vi "Graph - Multi-Y.vi"() -> ()   [LabVIEW 2020, in "Workspace MultiY Graph.lvlib"]
doc: "Sample numeric display item."
uses:
  MultiY Graph LLB.llb/Workspace MultiY Graph.lvlib
  MultiY Graph LLB.llb/cluster_Screen Item Settings.ctl
  MultiY Graph LLB.llb/cluster_Graph Scale Settings.ctl
  MultiY Graph LLB.llb/cluster_Graph Plot Settings.ctl
  NationalInstruments.VeriStand.SystemStorage
  MultiY Graph LLB.llb/XY Top level workspace graph data.ctl
  MultiY Graph LLB.llb/SystemStateRegEventRef.ctl
  MultiY Graph LLB.llb/Target State Info.ctl
  MultiY Graph LLB.llb/Target State.ctl
  MultiY Graph LLB.llb/enum_Display Template Handler Minimal To Widget Msg.ctl
  MultiY Graph LLB.llb/XY Dialog Msg to Control.ctl
  MultiY Graph LLB.llb/XY Dialog Msg Type.ctl
  MultiY Graph LLB.llb/XY Persistent Data.ctl
  MultiY Graph LLB.llb/XY Graph Properties.ctl
  MultiY Graph LLB.llb/XY Plot Properties.ctl
  MultiY Graph LLB.llb/XY Scale Properties.ctl
  MultiY Graph LLB.llb/XY Scale Precision.ctl
  MultiY Graph LLB.llb/XY Scale Format.ctl
  MultiY Graph LLB.llb/UDP Data.ctl
  MultiY Graph LLB.llb/Update Rate.ctl
  MultiY Graph LLB.llb/XY References.ctl
  MultiY Graph LLB.llb/enum_Display Template Handler Minimal To Workspace.ctl
  MultiY Graph LLB.llb/WorkspaceAPI.ctl
  MultiY Graph LLB.llb/SystemStateEventRef.ctl
  MultiY Graph LLB.llb/XY Control Msg to Dialog.ctl
  MultiY Graph LLB.llb/Net Event Data Ref.ctl
  MultiY Graph LLB.llb/Net Event Data.ctl
  MultiY Graph LLB.llb/Net Event.ctl
  MultiY Graph LLB.llb/UDPChannelStreamSession.ctl
  MultiY Graph LLB.llb/UDP Queue Data.ctl
  MultiY Graph LLB.llb/UDP Action State.ctl
  MultiY Graph LLB.llb/Graph Update Queue Data.ctl
  MultiY Graph LLB.llb/Graph Update Action State.ctl
  MultiY Graph LLB.llb/UDP Stream Configuration.ctl
  MultiY Graph LLB.llb/SystemState.ctl
  MultiY Graph LLB.llb/NI_VS Workspace ExecutionAPI.lvlib
  NationalInstruments.VeriStand.ClientAPI
  MultiY Graph LLB.llb/NI_VS UI Tree Alias Browser.lvlib
panel:
  in  "NIVS.Workspace Event":refnum<event-registration>
  in  "NIVS.System Definition Root":refnum<k24>
  in  "NIVS.Gateway IP Address":string
  out "Label":string="Waveform Graph"
  out "Graph":cluster{"X":dbl[], "Y":dbl[]}[](graph)
  in  "Item.Data":T1
  out "Y.Autoscale":bool
  in  "Y.Scale.Once":bool
  in  "Y.Scale.Auto":bool
  out "X.Autoscale":bool
  in  "X.Scale.Once":bool
  in  "X.Scale.Auto":bool
  in  "Legend":bool
  in  "Setup":bool
  in  "Hold":bool
  # "Autoscale X"
  # "Autoscale Y"
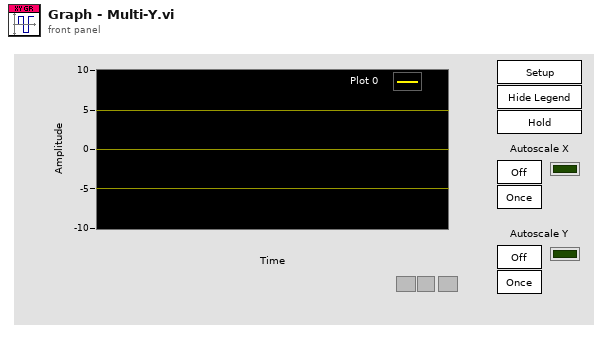
[diagram p1: front panel]
types:
  T1 = typedef "cluster_Screen Item Settings.ctl" = cluster{"Template VI":string, "Position X":i32, "Position Y":i32, "Custom":string, "Show Title Bar":bool, "ID":i32, "Always On Top":bool, "Allow Resize":bool, "Allow Minimize":bool, "Allow Close":bool, "Size to Screen":bool, "Screen.ID":i32, "State":enum16{"Normal", "New"}, "Title":string, "Window Bounds":cluster{"[0]":i16, "[1]":i16, "[2]":i16, "[3]":i16}, "Channel Ref":u64, "Unit":string, "Default Units?":bool, "Flash Limit?":bool, "Color 1":u32, "Color 2":u32, "Color 3":u32, "Color 4":u32, "Bck Color":u32, "Fore Color":u32, "Limit 1":dbl, "Limit 2":dbl, "Limit 3":dbl, "Limit 4":dbl, "Limit Mode 1":i32, "Limit Mode 2":i32, "Limit Mode 3":i32, "Limit Mode 4":i32, "Scale Precision":i32, "Scale Min":dbl, "Scale Max":dbl, "Format":i32, "Precision":i32, "Background Type":i32, "IDs":i32[], "Units":string[], "Labels":string[], "Scale Factor":dbl, "Scale Offset":dbl, "YScale Index":u32[], "XScale":T2, "YScales":T2[], "Plots":T3[], "Update Period":dbl, "History Length":dbl, "My.Ref":refnum<vi>, "Is Control?":bool, "Channel Paths":string[], "Custom Data":variant}
  T2 = typedef "cluster_Graph Scale Settings.ctl" = cluster{"Format":u8, "Precision":u8, "Fit":u8, "Label":string, "Use Default Label":bool, "Label Visible":bool, "Min":dbl, "Max":dbl}
  T3 = typedef "cluster_Graph Plot Settings.ctl" = cluster{"Bar Style":u8, "Fill To":i16, "Fill/PtColor":u32, "Line Style":u8, "Line Width":u8, "Color":u32, "Interp":u8, "Point Style":u8}
  T4 = typedef "Workspace MultiY Graph.lvlib/UDP Action State.ctl" = enum16{"Idle", "Open", "Acquire", "Send", "Close"}
  T5 = typedef "Workspace MultiY Graph.lvlib/UDP Stream Configuration.ctl" = cluster{"net address":u32, "Port":u16, "Channel IDs":i32[], "Packet IDs":i32[], "max packet size":i32, "Graph Buffer Size":i32, "Decimation":i32, "UDP Buffer Size":u32, "ByteOrder":i32}
  T6 = cluster{"connection ID":refnum<k16>, "UDP Stream Configuration":T5, "Graph Buffer":cluster{"X":dbl[], "Y":dbl[]}[], "Dynamic VI Refs":refnum<vi>[]}
  T7 = typedef "Workspace MultiY Graph.lvlib/Graph Update Action State.ctl" = enum16{"Active", "Change Rate", "Inactive"}
  T8 = typedef "Workspace MultiY Graph.lvlib/Graph Update Queue Data.ctl" = cluster{"Graph Update Action State":T7, "Data":variant}
  T9 = typedef "Workspace MultiY Graph.lvlib/UDP Queue Data.ctl" = cluster{"UDP Action State":T4, "Data":variant}
  T10 = typedef "Workspace MultiY Graph.lvlib/XY Top level workspace graph data.ctl" = cluster{"Custom Data":variant, "EventRegs":cluster{"SystemChange":T11, "WorkspaceState":refnum<event-registration>, "Graph":refnum<event-registration>, "Wks&Dialog&Periodic":refnum<event-registration>}, "References":T12, "Persistent Data":T13, "System":cluster{"To Workspace":refnum<user-event>, "From Workspace":refnum<user-event>, "NIVS helper":refnum<vi>, "Gtwy":string, "Root":refnum<k24>, "Workspace":T21, "SystemStateRefs":T22, "Connected?":bool, "FromDialog":refnum<user-event>, "ErrFlag":bool, "New":bool, "ErrState":string, "Save":bool, "Hold":bool, "Periodic":refnum<user-event>, "ToDialog":refnum<user-event>, "DialogEventReg":refnum<event-registration>, "UseSavedWidth":bool, "TreeBrowserEventReg":refnum<event-registration>, "UDPChannelStreamSession":T23, "Valid Channels?":bool, "Update Graph":refnum<user-event>, "UDP Queue":refnum<queue>, "Graph Update Queue":refnum<queue>}, "GraphData":cluster{"X":dbl[], "Y":dbl[]}[], "UDP Stream Active?":bool}
  T11 = typedef "NI_VS Workspace ExecutionAPI.lvlib/SystemStateRegEventRef.ctl" = refnum<event-registration>
  T12 = typedef "Workspace MultiY Graph.lvlib/XY References.ctl" = cluster{"X.Scale.Auto":refnum<vi>, "Y.Scale.Auto":refnum<vi>, "X.Scale.Once":refnum<vi>, "Y.Scale.Once":refnum<vi>, "LegendVis":refnum<vi>, "Graph":refnum<vi>}
  T13 = typedef "Workspace MultiY Graph.lvlib/XY Persistent Data.ctl" = cluster{"Label":string, "Graph Props":T14, "UDP Data":T19}
  T14 = typedef "Workspace MultiY Graph.lvlib/XY Graph Properties.ctl" = cluster{"Plots":T15[], "Legend:Number of Rows":u32, "Scale Properties":T16, "Legend:Visible":bool, "BgColor":u32, "Last Plot Width":u32, "Resize":bool}
  T15 = typedef "Workspace MultiY Graph.lvlib/XY Plot Properties.ctl" = cluster{"Bar Plot Style":u8, "Digital Line Style":u8, "Digital Transition Location":u8, "Digital Transition Type":u8, "Fill To":i16, "Fill/Point Color":u32, "Label Format":u8, "Line Style":u8, "Line Width":u8, "Plot Color":u32, "Plot Interpolation":u8, "Point Style":u8, "Visible":bool, "X Scale Index":u32, "Y Scale Index":u32}
  T16 = typedef "Workspace MultiY Graph.lvlib/XY Scale Properties.ctl" = cluster{"X.Auto":bool, "X.Min":dbl, "X.Max":dbl, "X.IgnoreTS":bool, "X.Precision":T17, "X.Label:":string, "X.LabelVis":bool, "X.DefLabel":bool, "Y.Auto":bool, "Y.Min":dbl, "Y.Max":dbl, "Y.Format":T18, "Y.Precision:":T17, "Y.Label:":string, "Y.LabelVis":bool, "Y.DefLabel":bool, "X.Format":T18}
  T17 = typedef "Workspace MultiY Graph.lvlib/XY Scale Precision.ctl" = u8
  T18 = typedef "Workspace MultiY Graph.lvlib/XY Scale Format.ctl" = u8
  T19 = typedef "Workspace MultiY Graph.lvlib/UDP Data.ctl" = cluster{"Decimation":i32, "UDP Buffer Size":u32, "History Length":dbl, "Update Rate":T20, "Channel Paths":string[], "Channel Names":string[]}
  T20 = typedef "Workspace MultiY Graph.lvlib/Update Rate.ctl" = enum8{"15 Hz", "10 Hz", "5 Hz", "4 Hz", "3 Hz", "2 Hz", "1 Hz", "0.5 Hz"}
  T21 = typedef "NI_VS Workspace ExecutionAPI.lvlib/WorkspaceAPI.ctl" = refnum<k24>
  T22 = typedef "NI_VS Workspace ExecutionAPI.lvlib/SystemStateEventRef.ctl" = cluster{"CustDatRef":refnum<user-event>, "EvtRef":refnum<k27>, "Target State User Event":refnum<user-event>}
  T23 = typedef "NI_VS Workspace ExecutionAPI.lvlib/UDPChannelStreamSession.ctl" = refnum<k24>
  T24 = cluster{"connection ID":refnum<k16>, "UDP Stream Configuration out":T5, "Array Out":cluster{"X":dbl[], "Y":dbl[]}[], "Dynamic VI Refs":refnum<vi>[]}
  T25 = typedef "Workspace MultiY Graph.lvlib/XY Control Msg to Dialog.ctl" = enum16{"Stop", "Connecting", "Disconnecting"}
  T26 = typedef "enum_Display Template Handler Minimal To Workspace.ctl" = cluster{"Operation":enum16{"SetCustomData", "DeleteItem"}, "Data":variant}
  T27 = cluster{"SystemChange":T11, "WorkspaceState":refnum<event-registration>, "Graph":refnum<event-registration>, "Wks&Dialog&Periodic":refnum<event-registration>}
  T28 = typedef "enum_Display Template Handler Minimal To Widget Msg.ctl" = enum16{"Stop", "LaunchConfigDialog"}
  T29 = typedef "Workspace MultiY Graph.lvlib/XY Dialog Msg Type.ctl" = enum16{"Update", "Delete"}
  T30 = typedef "NI_VS Workspace ExecutionAPI.lvlib/SystemState.ctl" = u8
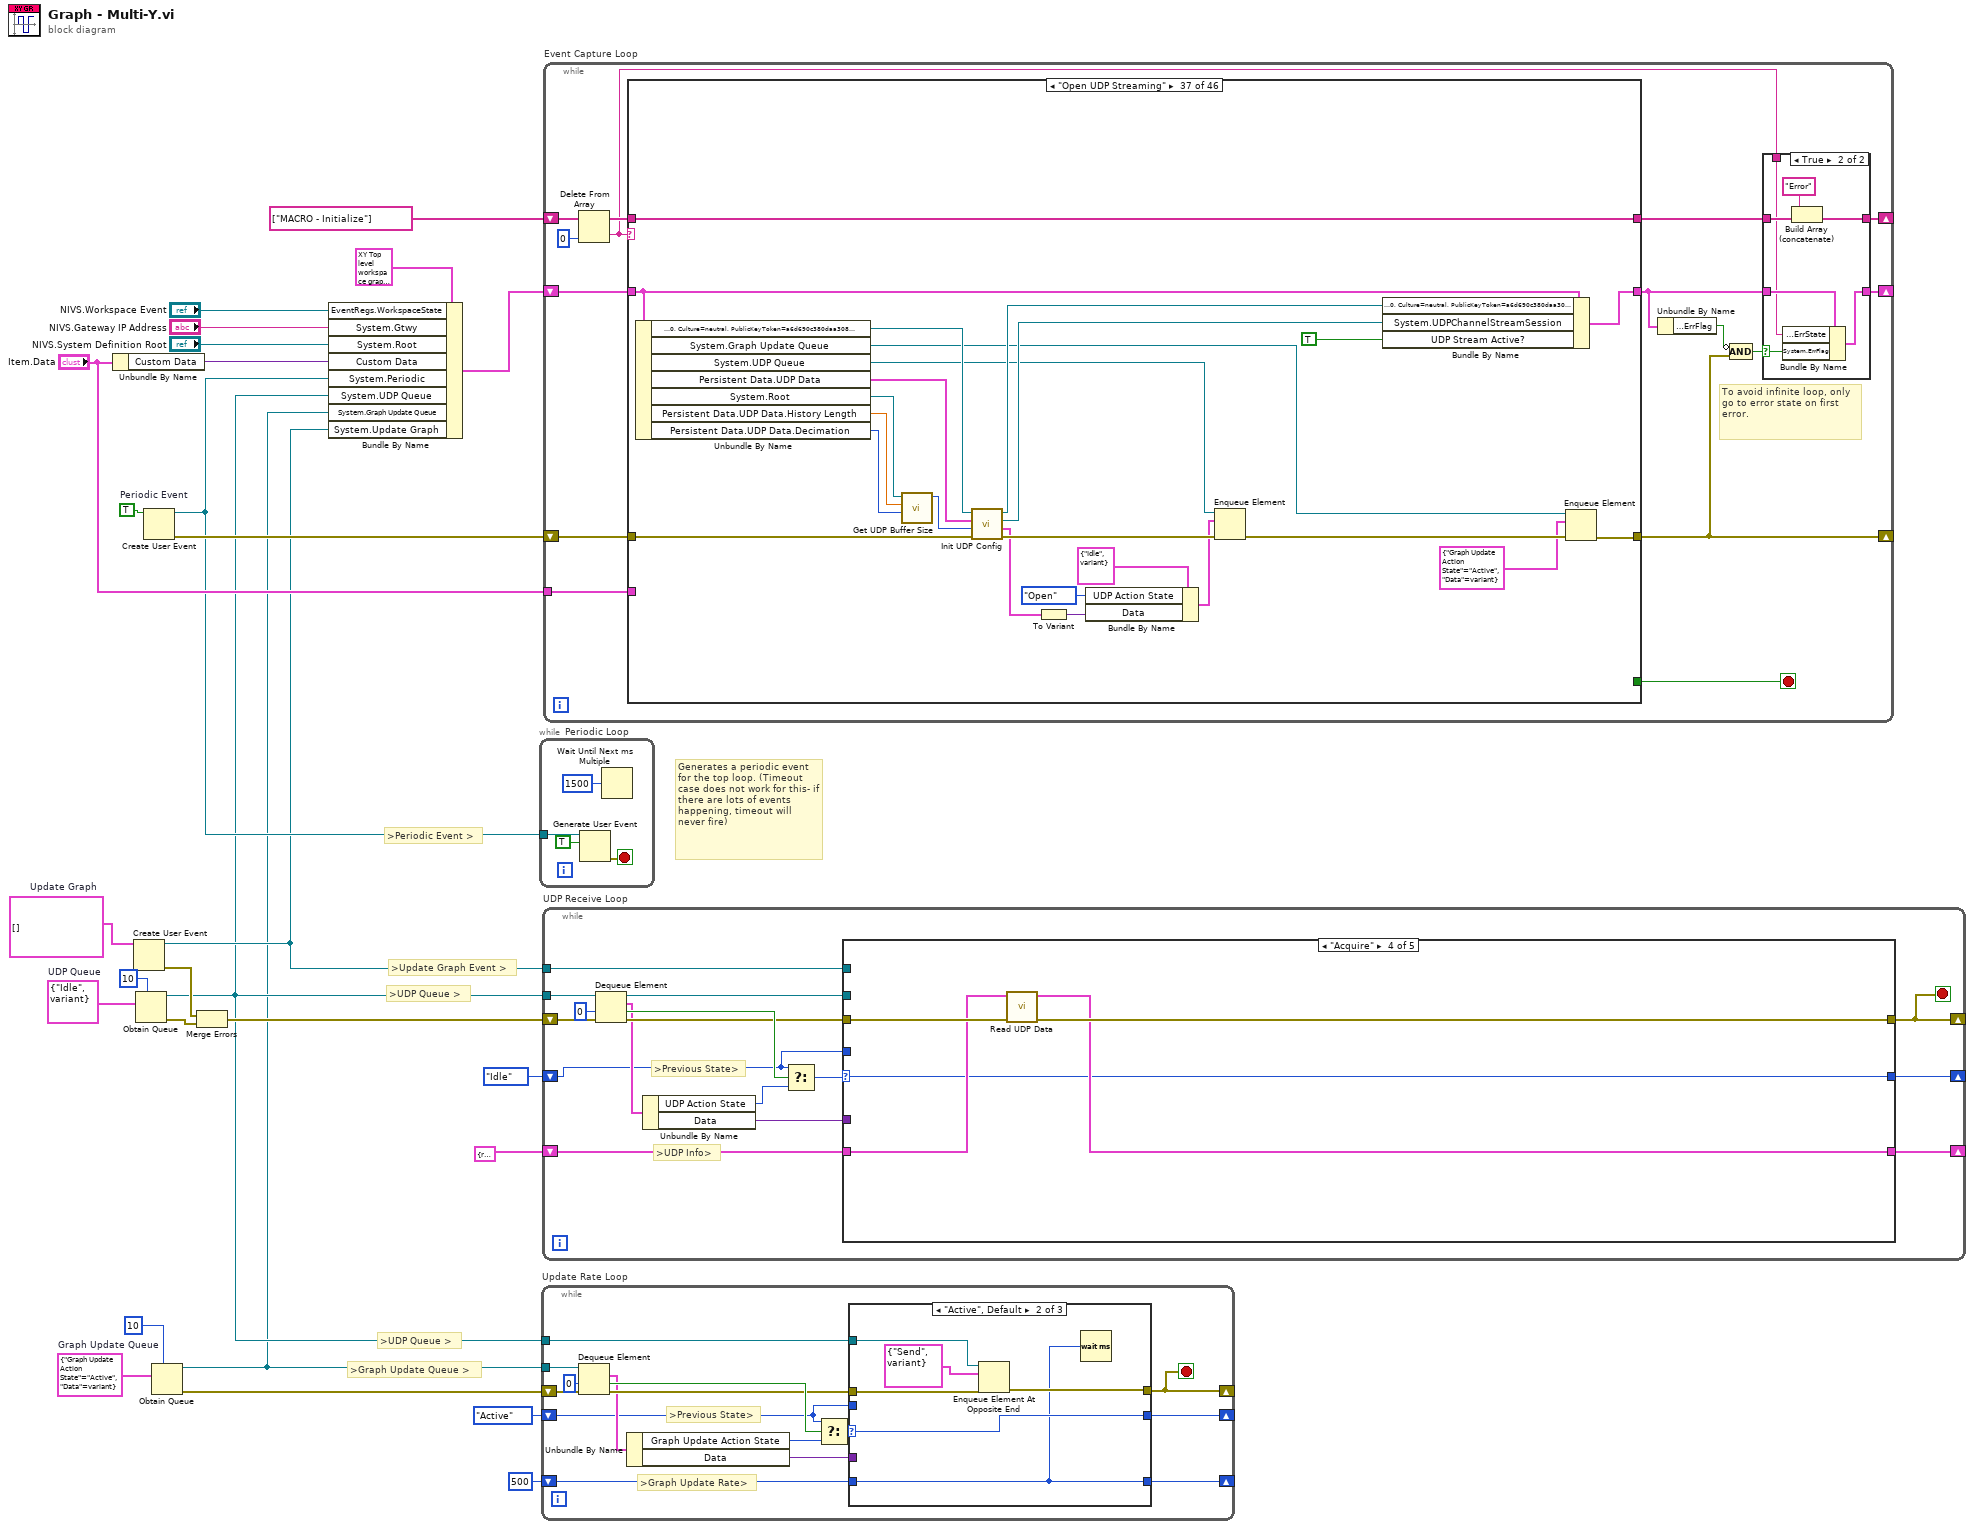
[diagram p0: block diagram]
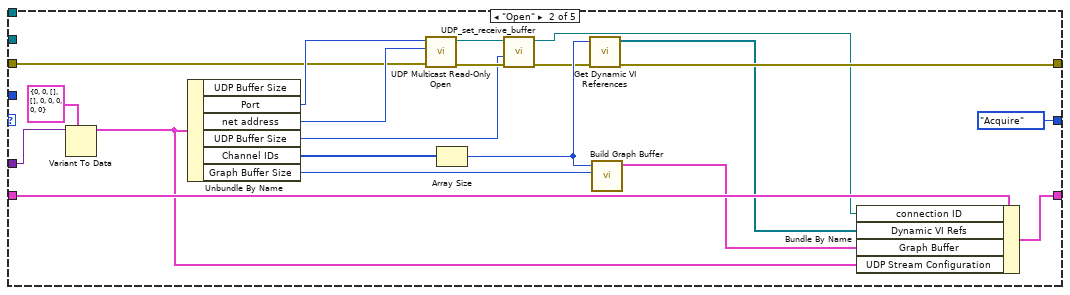
[diagram p3: hidden frame]
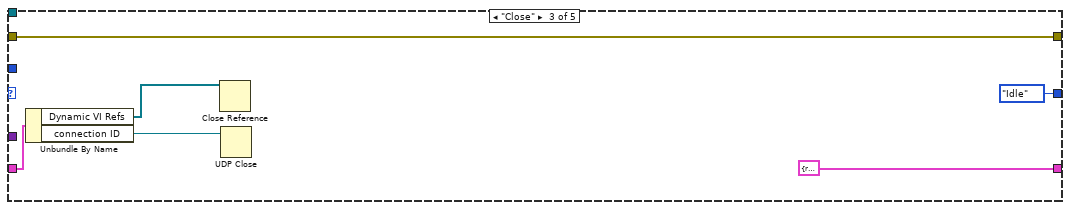
[diagram p4: hidden frame]
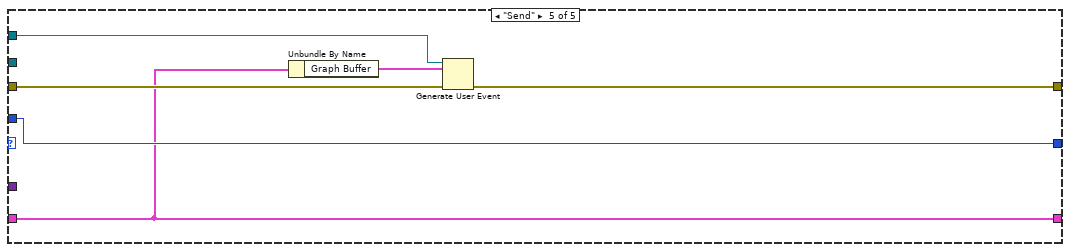
[diagram p5: hidden frame]
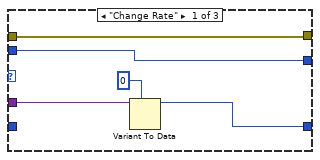
[diagram p6: hidden frame]
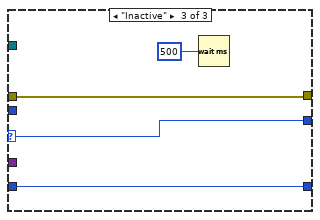
[diagram p7: hidden frame]
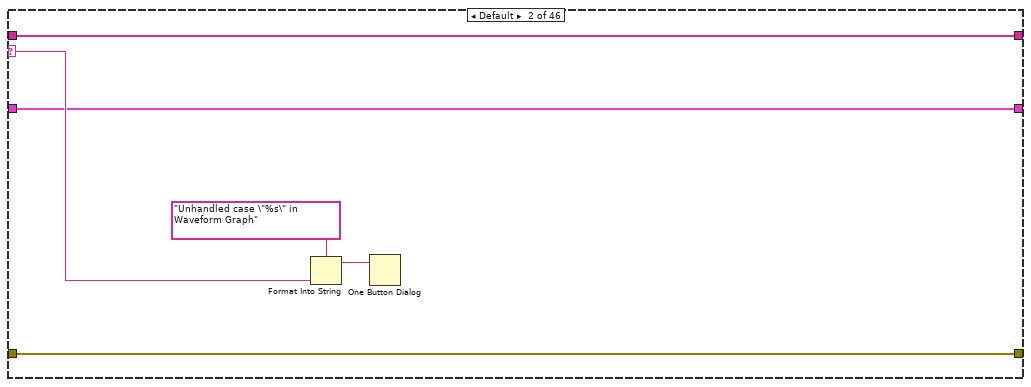
[diagram p10: hidden frame]
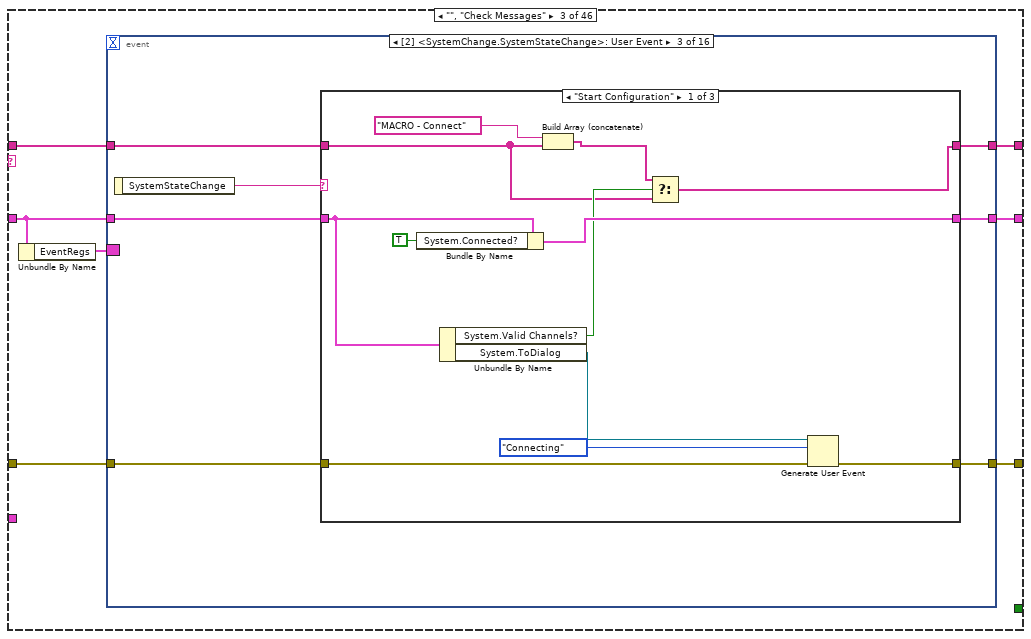
[diagram p11: hidden frame]
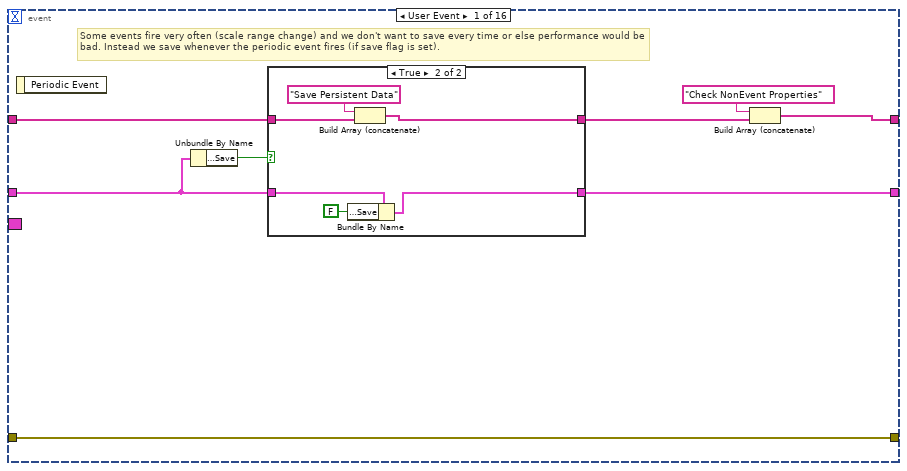
[diagram p12: hidden frame]
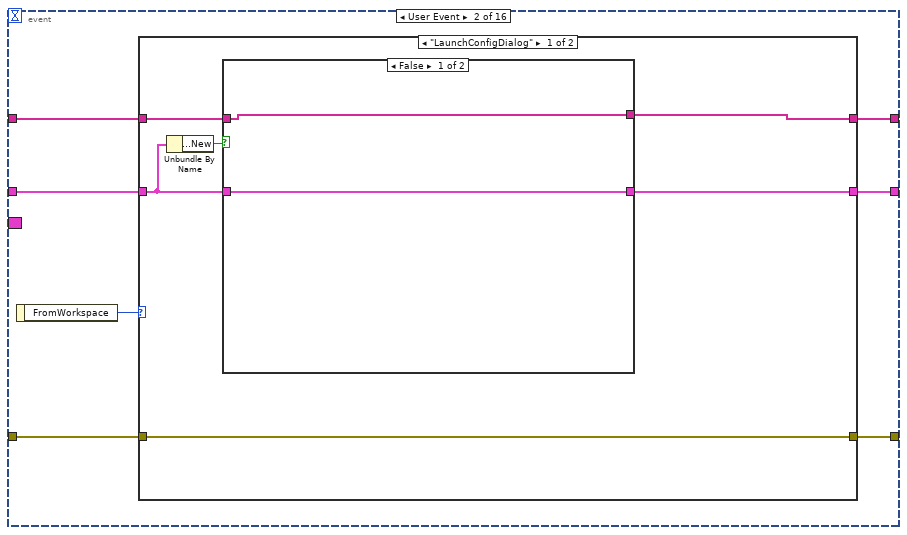
[diagram p14: hidden frame]
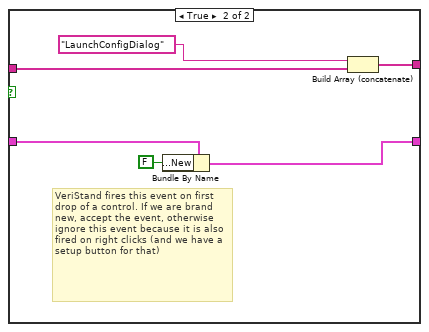
[diagram p15: hidden frame]
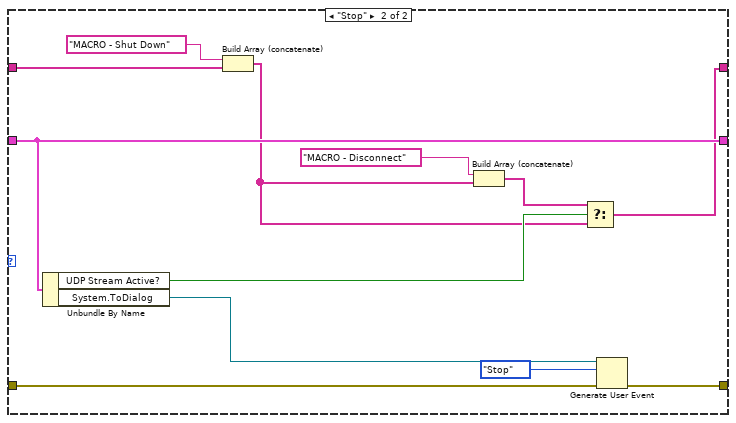
[diagram p16: hidden frame]
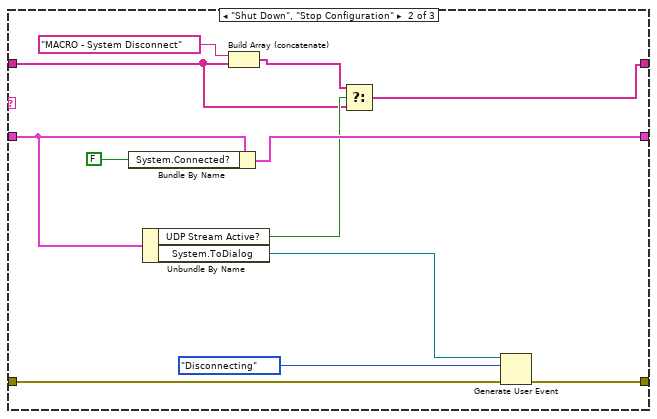
[diagram p17: hidden frame]
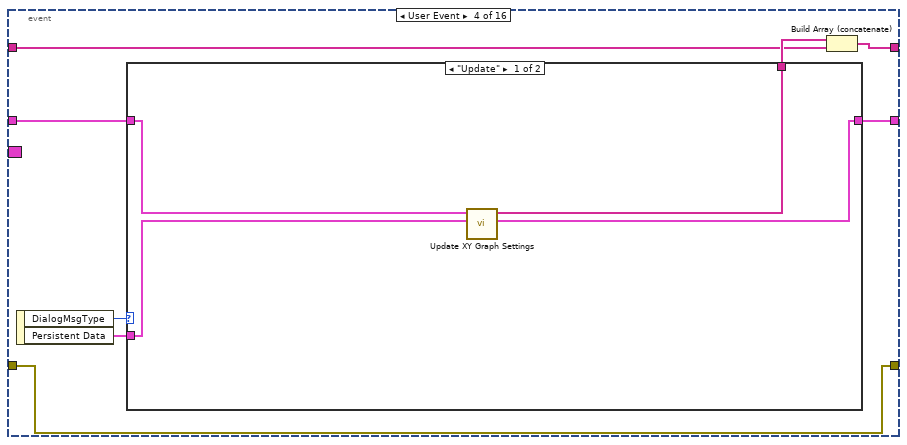
[diagram p19: hidden frame]
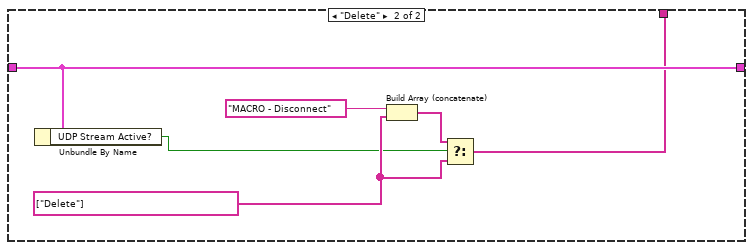
[diagram p20: hidden frame]
diagram:
  w13 = T8 {"Graph Update Action State"=enum."Active", "Data"=variant}  # Graph Update Queue
  w15 = T9 {"UDP Action State"=enum."Idle", "Data"=variant}  # UDP Queue
  w16 = cluster{"X":dbl[], "Y":dbl[]}[] []  # Update Graph
  w18 = TRUE  # Periodic Event
  # ">UDP Queue >"
  # ">Update Graph Event >"
  # ">Periodic Event >"
  # ">Graph Update Queue >"
  # ">UDP Queue >"
  # "Generates a periodic event for the top loop. (Timeout case does not work for this- if there are lots of events happening, timeout will never fire)"
  n1 = Unbundle By Name("Item.Data") -> ("Custom Data"=w26:variant)
  n2 = Create User Event(user event datatype=w16) -> (user event=w14:refnum<user-event>, error out=w9:errorcluster)  [unwired: 1 in]
  n3 = Obtain Queue(max queue size (-1, unlimited)=10, element data type=w15) -> (queue out=w6:refnum<queue>, error out=w10:errorcluster)  [unwired: 3 in, 1 out]
  n4 = Create User Event(user event datatype=w18) -> (user event=w17:refnum<user-event>, error out=w19:errorcluster)  [unwired: 1 in]
  n5 = Obtain Queue(max queue size (-1, unlimited)=10, element data type=w13) -> (queue out=w3:refnum<queue>, error out=w11:errorcluster)  [unwired: 3 in, 1 out]
  n6 = Merge Errors(w9, w10) -> (w8:errorcluster)
  n7 = Bundle By Name(cluster=T10 {"Custom Data"=variant, "EventRegs"={"SystemChange"=refnum, "WorkspaceState"=refnum, "Graph"=refnum, "Wks&Dialog&Periodic"=refnum}, "References"={"X.Scale.Auto"=refnum, "Y.Scale.Auto"=refnum, "X.Scale.Once"=refnum, "Y.Scale.Once"=refnum, "LegendVis"=refnum, "Graph"=refnum}, "Persistent Data"={"Label"="", "Graph Props"={"Plots"=[], "Legend:Number of Rows"=0, "Scale Properties"={"X.Auto"=FALSE, "X.Min"=0.0, "X.Max"=0.0, "X.IgnoreTS"=FALSE, "X.Precision"=0, "X.Label:"="", "X.LabelVis"=FALSE, "X.DefLabel"=FALSE, "Y.Auto"=FALSE, "Y.Min"=0.0, "Y.Max"=0.0, "Y.Format"=0, "Y.Precision:"=0, "Y.Label:"="", "Y.LabelVis"=FALSE, "Y.DefLabel"=FALSE, "X.Format"=0}, "Legend:Visible"=FALSE, "BgColor"=0, "Last Plot Width"=0, "Resize"=FALSE}, "UDP Data"={"Decimation"=0, "UDP Buffer Size"=0, "History Length"=0.0, "Update Rate"=enum."15 Hz", "Channel Paths"=[], "Channel Names"=[]}}, "System"={"To Workspace"=refnum, "From Workspace"=refnum, "NIVS helper"=refnum, "Gtwy"="", "Root"=refnum, "Workspace"=refnum, "SystemStateRefs"={"CustDatRef"=refnum, "EvtRef"=refnum, "Target State User Event"=refnum}, "Connected?"=FALSE, "FromDialog"=refnum, "ErrFlag"=FALSE, "New"=FALSE, "ErrState"="", "Save"=FALSE, "Hold"=FALSE, "Periodic"=refnum, "ToDialog"=refnum, "DialogEventReg"=refnum, "UseSavedWidth"=FALSE, "TreeBrowserEventReg"=refnum, "UDPChannelStreamSession"=refnum, "Valid Channels?"=FALSE, "Update Graph"=refnum, "UDP Queue"=refnum, "Graph Update Queue"=refnum}, "GraphData"=[], "UDP Stream Active?"=FALSE} ("Waveform Graph Data"), "EventRegs.WorkspaceState"="NIVS.Workspace Event", "System.Gtwy"="NIVS.Gateway IP Address", "System.Root"="NIVS.System Definition Root", "Custom Data"=w26, "System.Periodic"=w17, "System.UDP Queue"=w6, "System.Graph Update Queue"=w3, "System.Update Graph"=w14) -> (w21:T10)
  n8 = while "Periodic Loop" {
    tunnel: w17 -> [w30]
    stop <- w29 stop-if-true
    n9 = Generate User Event(user event=w30, event data cluster=TRUE ("event data")) -> (error out=w29:errorcluster)  [unwired: 2 in, 1 out]
    n10 = Wait Until Next ms Multiple(millisecond multiple=u32 1500) -> ()  [unwired: 1 out]
  }
  n11 = while "Update Rate Loop" {
    tunnel: w3 -> [w45]
    shift-right: [w39] -> _
    shift-left: w11 -> [w46]
    shift-right: [w41] -> _
    shift-left: Graph_Update_Action_State."Active" ("Graph Update Action State") -> [w33]
    tunnel: w6 -> [w38]
    shift-right: [w34] -> _
    shift-left: u32 500 ("element") -> [w32]
    stop <- w39 stop-if-true
    # ">Previous State>"
    # ">Graph Update Rate>"
    n12 = Dequeue Element(queue=w45, timeout in ms (-1)=0, error in (no error)=w46) -> (element=w37:T8, timed out?=w43:bool, error out=w40:errorcluster)  [unwired: 1 out]
    n13 = Unbundle By Name(w37) -> ("Graph Update Action State"=w36:T7, "Data"=w35:variant)
    n14 = Select(t=w33, s=w43, f=w36) -> (s? t:f=w42:T7)
    n15 = case shown="\"Active\", Default" w42 {
      selector: w42 -> [_ w57 w61]
      tunnel: [w47 w57 w61] -> w41
      tunnel: w40 -> [w51 w56 w60]
      tunnel: [w51 w53 w60] -> w39
      tunnel: w38 -> [_ w55 _]
      tunnel: w35 -> [w50 _ _]
      tunnel: [w48 w52 w58] -> w34
      tunnel: w33 -> [w47 _ _]
      tunnel: w32 -> [_ w52 w58]
      frame "Change Rate" {
        n16 = Variant To Data(type=u32 0 ("element"), Variant=w50) -> (data=w48:u32)  [unwired: 1 in, 1 out]
      }
      frame "Active", Default {
        n17 = Enqueue Element At Opposite End(queue=w55, element=T9 {"UDP Action State"=enum."Send", "Data"=variant} ("notification"), error in (no error)=w56) -> (error out=w53:errorcluster)  [unwired: 1 in, 2 out]
        n18 = Wait (ms)(milliseconds to wait=w52) -> ()  [unwired: 1 out]
      }
      frame "Inactive" {
        n19 = Wait (ms)(milliseconds to wait=u32 500) -> ()  [unwired: 1 out]
      }
    }
  }
  n20 = while "UDP Receive Loop" {
    tunnel: w6 -> [w76]
    shift-right: [w70] -> _
    shift-left: w8 -> [w77]
    shift-right: [w72] -> _
    shift-left: UDP_Action_State."Idle" ("UDP Action State") -> [w63]
    shift-right: [w68] -> _
    shift-left: T6 {"connection ID"=refnum, "UDP Stream Configuration"={"net address"=0, "Port"=0, "Channel IDs"=[], "Packet IDs"=[], "max packet size"=0, "Graph Buffer Size"=0, "Decimation"=0, "UDP Buffer Size"=0, "ByteOrder"=0}, "Graph Buffer"=[], "Dynamic VI Refs"=[]} -> [w69]
    tunnel: w14 -> [w62]
    stop <- w70 stop-if-true
    # ">UDP Info>"
    # ">Previous State>"
    n21 = Dequeue Element(queue=w76, timeout in ms (-1)=0, error in (no error)=w77) -> (queue out=w75:refnum<queue>, element=w65:T9, timed out?=w73:bool, error out=w71:errorcluster)
    n22 = Unbundle By Name(w65) -> ("UDP Action State"=w66:T4, "Data"=w64:variant)
    n23 = Select(t=w63, s=w73, f=w66) -> (s? t:f=w67:T4)
    n24 = case shown="\"Acquire\"" w67 {
      selector: w67 -> [w80 _ _ w107 _]
      tunnel: w71 -> [w79 w88 w102 w111 w114]
      tunnel: [w79 w93 w102 w110 w113] -> w70
      tunnel: w75 -> [_ _ _ _ _]
      tunnel: [w80 UDP_Action_State."Acquire" ("UDP Action State") UDP_Action_State."Idle" ("UDP Action State") w107 w117] -> w72
      tunnel: w69 -> [w78 w97 w105 w109 w112]
      tunnel: [w78 w96 T24 {"connection ID"=refnum, "UDP Stream Configuration out"={"net address"=0, "Port"=0, "Channel IDs"=[], "Packet IDs"=[], "max packet size"=0, "Graph Buffer Size"=0, "Decimation"=0, "UDP Buffer Size"=0, "ByteOrder"=0}, "Array Out"=[], "Dynamic VI Refs"=[]} w108 w112] -> w68
      tunnel: w64 -> [_ w91 _ _ _]
      tunnel: w63 -> [_ _ _ _ w117]
      tunnel: w62 -> [_ _ _ _ w115]
      frame "Idle", Default {
      }
      frame "Open" {
        n25 = Variant To Data(type=T5 {"net address"=0, "Port"=0, "Channel IDs"=[], "Packet IDs"=[], "max packet size"=0, "Graph Buffer Size"=0, "Decimation"=0, "UDP Buffer Size"=0, "ByteOrder"=0} ("UDP Stream Configuration out"), Variant=w91) -> (data=w89:T5)  [unwired: 1 in, 1 out]
        n26 = Unbundle By Name(w89) -> ("Port"=w100:u16, "net address"=w99:u32, "UDP Buffer Size"=w81:u32, "Channel IDs"=w95:i32[], "Graph Buffer Size"=w98:i32)  [unwired: 1 out]
        n27 = call "UDP Multicast Read-Only Open.vi"("error in (no error)"=w88, "multicast addr"=w99, "port"=w100) -> ("error out"=w85:errorcluster, "connection ID"=w84:refnum<k16>)  [unwired: 6 in, 1 out]
        n28 = Array Size(array=w95) -> (size(s)=w94:i32)
        n29 = call "UDP_set_receive_buffer.vi"("error in (no error)"=w85, "Receive Buffer Size"=w81, "connection ID"=w84) -> ("error out"=w82:errorcluster, "connection ID out"=w83:refnum<k16>)  [unwired: 6 in]
        n30 = call "Get Dynamic VI References.vi"("error in (no error)"=w82, "Channel Count"=w94) -> ("error out"=w93:errorcluster, "Dynamic VI References"=w92:refnum<vi>[])  [unwired: 8 in]
        n31 = call "Build Graph Buffer.vi"("Graph Buffer Size"=w98, "Channel Count"=w94) -> ("Graph Buffer out"=w86:cluster{dbl[], dbl[]}[])  [unwired: 9 in]
        n32 = Bundle By Name(cluster=w97, "connection ID"=w83, "Dynamic VI Refs"=w92, "Graph Buffer"=w86, "UDP Stream Configuration"=w89) -> (w96:T6)
      }
      frame "Close" {
        n33 = Unbundle By Name(w105) -> ("Dynamic VI Refs"=w104:refnum<vi>[], "connection ID"=w103:refnum<k16>)
        n34 = Close Reference(reference=w104) -> ()  [unwired: 1 in, 1 out]
        n35 = UDP Close(connection ID=w103) -> ()  [unwired: 1 in, 2 out]
      }
      frame "Acquire" {
        n36 = call "Read UDP Data.vi"("error in (no error)"=w111, "UDP Cluster in"=w109) -> ("error out"=w110:errorcluster, "UDP Cluster out"=w108:T6)  [unwired: 8 in]
      }
      frame "Send" {
        n37 = Unbundle By Name(w112) -> ("Graph Buffer"=w116:cluster{"X":dbl[], "Y":dbl[]}[])
        n38 = Generate User Event(user event=w115, event data cluster=w116, error in=w114) -> (error out=w113:errorcluster)  [unwired: 1 in, 1 out]
      }
    }
  }
  n39 = while "Event Capture Loop" {
    shift-right: [w126] -> _
    shift-left: string[] ["MACRO - Initialize"] -> [w132]
    shift-right: [w119] -> _
    shift-left: w19 -> [w125]
    shift-right: [w123] -> _
    shift-left: w21 -> [w128]
    tunnel: "Item.Data" -> [w127]
    stop <- w130 stop-if-true
    # "To avoid infinite loop, only go to error state on first error."
    n40 = Delete From Array(array=w132, index=0) -> (deleted portion=w118:string, array with subset deleted=w131:string[])  [unwired: 1 in]
    n41 = case shown="\"Open UDP Streaming\"" w118 {
      selector: w118 -> [_ w149 _ _ _ _ _ _ _ _ _ _ _ _ _ _ _ _ _ _ _ _ _ _ _ _ _ _ _ _ _ _ _ _ _ _ _ _ _ _ _ _ _ _ _ _]
      tunnel: [w142 w145 w157 string[] ["MACRO - Disconnect"] w440 w448 w450 w459 w460 w470 w482 w485 w489 w507 w530 w541 w552 w585 w619 w635 w656 w681 w689 w699 w700 w704 w707 w714 w718 w723 w728 w733 w739 w755 w769 w772 w796 w797 w806 w809 w818 w823 w838 w847 w871 w889] -> w129
      tunnel: w131 -> [w142 w145 w156 _ w440 w448 w450 w459 w460 w470 w482 w485 w489 w507 w530 w541 w552 w585 w619 w635 w656 w681 w689 w699 w700 w704 w708 w715 w721 w724 w729 w736 w739 w755 w769 w772 w796 w797 w806 w809 w818 w827 w838 w846 w871 w889]
      tunnel: [_ _ _ _ _ _ _ _ _ _ _ _ _ _ _ _ _ _ _ _ _ _ _ _ TRUE _ _ _ _ _ _ _ _ _ _ _ _ _ _ _ _ _ _ _ _ _] -> w130
      tunnel: w125 -> [w144 w147 w154 w424 w436 w447 w452 w453 w466 w469 w473 w484 w488 w506 w529 w540 w547 w584 w618 w632 w658 w667 w688 w692 w702 w706 w711 w716 w720 w726 w731 w735 w738 w752 w766 w771 w794 w799 w805 w808 w821 w832 w837 w852 w869 w885]
      tunnel: [w144 w147 w153 errorcluster {"status"=FALSE, "code"=0, "source"=""} ("error constant") w439 w444 w451 w453 w464 w469 w472 w484 w488 w495 w517 w537 w548 w576 w615 w633 w658 w674 w685 w691 w702 w706 w711 w716 w720 w726 w731 w735 w738 w741 w758 w771 w787 w799 w800 w810 w821 w831 w837 w851 w865 w886] -> w119
      tunnel: w128 -> [w143 w146 w152 w426 w433 w446 w449 w458 w467 w468 w481 w483 w487 w499 w522 w539 w551 w583 w617 w634 w657 w684 w687 w698 w701 w705 w710 w713 w719 w725 w730 w734 w737 w751 w765 w770 w791 w798 w802 w807 w820 w829 w836 w842 w870 w879]
      tunnel: [w143 w146 w155 w426 w432 w445 w449 w457 w467 w468 w481 w483 w487 w498 w521 w539 w551 w583 w617 w634 w657 w684 w687 w698 w701 w705 w710 w713 w719 w725 w730 w734 w737 w750 w764 w770 w790 w798 w804 w811 w819 w828 w835 w844 w870 w873] -> w122
      tunnel: w127 -> [_ _ _ _ _ _ _ _ _ _ _ _ _ _ _ _ _ _ _ _ _ _ _ _ _ _ _ _ _ _ _ _ _ _ _ _ _ _ _ _ _ _ _ _ _ w875]
      frame "<------------------ System ------------------>" {
      }
      frame Default {
        n42 = Format Into String(format string="Unhandled case \"%s\" in Waveform Graph", w149) -> (resulting string=w150:string)  [unwired: 2 in, 1 out]
        n43 = One Button Dialog(message=w150) -> ()  [unwired: 1 in, 1 out]
      }
      frame "", "Check Messages" {
        n44 = Unbundle By Name(w152) -> ("EventRegs"=w151:T27)
        n45 = event shown="[2] <SystemChange.SystemStateChange>: User Event" {
          selector: w151 -> [_ _ _ _ _ _ _ _ _ _ _ _ _ _ _ _]
          dyn-events: _ -> [_ _ _ _ _ _ _ _ _ _ _ _ _ _ _ _]
          timeout: _ -> [_ _ _ _ _ _ _ _ _ _ _ _ _ _ _ _]
          tunnel: [w158 w174 w213 w246 w265 w286 w293 w300 w306 w316 w323 w335 w343 w354 w367 w380] -> w157
          tunnel: w156 -> [w165 w178 w212 w247 w264 w286 w293 w302 w314 w321 w328 w338 w349 w360 w367 w379]
          tunnel: [w164 w175 w211 w245 w263 w284 w289 w304 w308 w318 w325 w337 w341 w352 w362 w381] -> w155
          tunnel: w152 -> [w162 w176 w210 w244 w262 w281 w292 w304 w310 w319 w326 w331 w346 w357 w365 w382]
          tunnel: w154 -> [w161 w180 w208 w241 w260 w282 w291 w303 w313 w320 w327 w333 w348 w359 w366 w383]
          tunnel: [w161 w177 w209 w241 w261 w282 w290 w303 w312 w320 w327 w332 w347 w358 w366 w384] -> w153
          event User Event {
            # "Some events fire very often (scale range change) and we don't want to save every time or else performance would be bad. Instead we save whenever the periodic event fires (if save flag is set)."
            n46 = event-data() -> ()  [unwired: 1 in, 1 out]
            n47 = Unbundle By Name(w162) -> ("System.Save"=w163:bool)
            n48 = case shown="True" w163 {
              tunnel: w165 -> [w167 w170]
              tunnel: [w167 w168] -> w160
              tunnel: [w166 w171] -> w164
              tunnel: w162 -> [w166 w173]
              frame False {
              }
              frame True {
                n49 = Bundle By Name(cluster=w173, "System.Save"=FALSE) -> (w171:T10)
                n50 = Build Array (concatenate)("Save Persistent Data", w170) -> (w168:string[])
              }
            }
            n51 = Build Array (concatenate)("Check NonEvent Properties", w160) -> (w158:string[])
          }
          event User Event {
            n52 = event-data() -> ("FromWorkspace"=w179:T28)  [unwired: 1 in]
            n53 = case shown="\"LaunchConfigDialog\"" w179 {
              tunnel: w180 -> [w186 w203]
              tunnel: w178 -> [w185 w206]
              tunnel: [w186 w202] -> w177
              tunnel: w176 -> [w182 w204]
              tunnel: [w181 w204] -> w175
              tunnel: [w184 w195] -> w174
              frame "LaunchConfigDialog" {
                n54 = Unbundle By Name(w182) -> ("System.New"=w183:bool)
                n55 = case shown="False" w183 {
                  tunnel: w185 -> [w187 w194]
                  tunnel: [w187 w192] -> w184
                  tunnel: w182 -> [w188 w191]
                  tunnel: [w188 w190] -> w181
                  frame False {
                  }
                  frame True {
                    # "VeriStand fires this event on first drop of a control. If we are brand new, accept the event, otherwise ignore this event because it is also fired on right clicks (and we have a setup button for that)"
                    n56 = Bundle By Name(cluster=w191, "System.New"=FALSE) -> (w190:T10)
                    n57 = Build Array (concatenate)("LaunchConfigDialog", w194) -> (w192:string[])
                  }
                }
              }
              frame "Stop" {
                n58 = Unbundle By Name(w204) -> ("UDP Stream Active?"=w197:bool, "System.ToDialog"=w201:refnum<user-event>)
                n59 = Build Array (concatenate)("MACRO - Shut Down", w206) -> (w196:string[])
                n60 = Build Array (concatenate)("MACRO - Disconnect", w196) -> (w198:string[])
                n61 = Select(t=w198, s=w197, f=w196) -> (s? t:f=w195:string[])
                n62 = Generate User Event(user event=w201, event data cluster=XY_Control_Msg_to_Dialog."Stop" ("event data"), error in=w203) -> (error out=w202:errorcluster)  [unwired: 1 in, 1 out]
              }
            }
          }
          event User Event {
            n63 = event-data() -> ("SystemStateChange"=w207:string)  [unwired: 1 in]
            n64 = case shown="\"Start Configuration\"" w207 {
              tunnel: [w214 w226 w240] -> w213
              tunnel: w212 -> [w216 w227 w240]
              tunnel: [w224 w236 w239] -> w211
              tunnel: w210 -> [w219 w230 w239]
              tunnel: [w220 w231 w238] -> w209
              tunnel: w208 -> [w221 w232 w238]
              frame "Start Configuration" {
                n65 = Bundle By Name(cluster=w219, "System.Connected?"=TRUE) -> (w224:T10)
                n66 = Unbundle By Name(w219) -> ("System.Valid Channels?"=w217:bool, "System.ToDialog"=w223:refnum<user-event>)
                n67 = Build Array (concatenate)("MACRO - Connect", w216) -> (w215:string[])
                n68 = Select(t=w215, s=w217, f=w216) -> (s? t:f=w214:string[])
                n69 = Generate User Event(user event=w223, event data cluster=XY_Control_Msg_to_Dialog."Connecting" ("event data"), error in=w221) -> (error out=w220:errorcluster)  [unwired: 1 in, 1 out]
              }
              frame "Shut Down", "Stop Configuration" {
                n70 = Bundle By Name(cluster=w230, "System.Connected?"=FALSE) -> (w236:T10)
                n71 = Unbundle By Name(w230) -> ("UDP Stream Active?"=w229:bool, "System.ToDialog"=w234:refnum<user-event>)
                n72 = Build Array (concatenate)("MACRO - System Disconnect", w227) -> (w228:string[])
                n73 = Select(t=w228, s=w229, f=w227) -> (s? t:f=w226:string[])
                n74 = Generate User Event(user event=w234, event data cluster=XY_Control_Msg_to_Dialog."Disconnecting" ("event data"), error in=w232) -> (error out=w231:errorcluster)  [unwired: 1 in, 1 out]
              }
              frame Default {
              }
            }
          }
          event User Event {
            n75 = event-data() -> ("DialogMsgType"=w242:T29, "Persistent Data"=w243:T13)  [unwired: 1 in]
            n76 = case shown="\"Update\"" w242 {
              tunnel: w244 -> [w251 w258]
              tunnel: [w252 w258] -> w245
              tunnel: w243 -> [w250 _]
              tunnel: [w249 w254] -> w248
              frame "Update" {
                n77 = call "Update XY Graph Settings.vi"("Persistent Data"=w250, "Waveform Graph Data in"=w251) -> ("Waveform Graph Data out"=w252:T10, "State Array"=w249:string[])  [unwired: 8 in]
              }
              frame "Delete" {
                w256 = string[] ["Delete"]
                n78 = Unbundle By Name(w258) -> ("UDP Stream Active?"=w253:bool)
                n79 = Build Array (concatenate)("MACRO - Disconnect", w256) -> (w255:string[])
                n80 = Select(t=w255, s=w253, f=w256) -> (s? t:f=w254:string[])
              }
            }
            n81 = Build Array (concatenate)(w248, w247) -> (w246:string[])
          }
          event User Event {
            # "Workspace and/or project  is closing"
            n82 = event-data() -> ("Workspace Event"=w259:string)  [unwired: 1 in]
            n83 = case shown="\"Shut Down\"" w259 {
              tunnel: [w266 w280] -> w265
              tunnel: w264 -> [w277 w280]
              tunnel: [w271 w279] -> w263
              tunnel: w262 -> [w271 w279]
              tunnel: [w272 w278] -> w261
              tunnel: w260 -> [w273 w278]
              frame "Shut Down" {
                n84 = Unbundle By Name(w271) -> ("UDP Stream Active?"=w270:bool, "System.ToDialog"=w275:refnum<user-event>)
                n85 = Build Array (concatenate)("MACRO - Shut Down", w277) -> (w267:string[])
                n86 = Build Array (concatenate)("MACRO - System Disconnect", w267) -> (w268:string[])
                n87 = Select(t=w268, s=w270, f=w267) -> (s? t:f=w266:string[])
                n88 = Generate User Event(user event=w275, event data cluster=XY_Control_Msg_to_Dialog."Stop" ("event data"), error in=w273) -> (error out=w272:errorcluster)  [unwired: 1 in, 1 out]
              }
              frame Default {
              }
            }
          }
          event User Event {
            n89 = event-data() -> ("Update Graph"=w285:cluster{"X":dbl[], "Y":dbl[]}[])  [unwired: 1 in]
            n90 = Unbundle By Name(w281) -> ("System.Hold"=w283:bool)
            n91 = case shown="False" w283 {
              tunnel: w285 -> [w287 _]
              frame False {
                "Graph" <- w287
              }
              frame True {
              }
            }
            n92 = Bundle By Name(cluster=w281, "GraphData"=w285) -> (w284:T10)
          }
          event "Hold": Value Change {
            n93 = event-data() -> ("NewVal"=w288:bool)  [unwired: 1 in]
            n94 = case shown="False" w288 {
              tunnel: w292 -> [w298 _]
              tunnel: w291 -> [w297 w299]
              tunnel: [w296 w299] -> w290
              frame False {
                # "Graph was unheld. immediately refresh."
                n95 = Unbundle By Name(w298) -> ("References.Graph"=w295:refnum<vi>, "GraphData"=w294:cluster{"X":dbl[], "Y":dbl[]}[])
                n96 = property class="XYGraph (strict)"(reference=w295, error in=w297, "Value"=w294) -> (error out=w296:errorcluster)  [unwired: 1 out]
              }
              frame True {
                # "Graph held. The wfm data event case will not update the graph"
              }
            }
            n97 = Bundle By Name(cluster=w292, "System.Hold"=w288) -> (w289:T10)
          }
          event "Setup": Value Change {
            n98 = event-data() -> ()  [unwired: 1 in, 2 out]
            n99 = Build Array (concatenate)("LaunchConfigDialog", w302) -> (w300:string[])
          }
          event "Graph": Plot Attribute Change {
            # "Rather than figure out what changed exactly.. just read & save it all"
            n100 = event-data() -> ()  [unwired: 1 in, 1 out]
            n101 = Unbundle By Name(w310) -> ("References.Graph"=w311:refnum<vi>)
            n102 = call "Get XY Plot Properties from Graph.vi"("error in (no error)"=w313, "Graph"=w311) -> ("error out"=w312:errorcluster, "Plots"=w309:T15[], "Legend:Number of Rows"=w307:u32)  [unwired: 7 in]
            n103 = Build Array (concatenate)("Save Persistent Data", w314) -> (w306:string[])
            n104 = Bundle By Name(cluster=w310, "Persistent Data.Graph Props.Legend:Number of Rows"=w307, "Persistent Data.Graph Props.Plots"=w309) -> (w308:T10)
          }
          event "X.Scale.Auto": Value Change {
            n105 = event-data() -> ("NewVal"=w317:bool)  [unwired: 1 in]
            n106 = Bundle By Name(cluster=w319, "Persistent Data.Graph Props.Scale Properties.X.Auto"=w317) -> (w318:T10)
            n107 = Build Array (concatenate)(string[] ["Set Autoscale X", "Save Persistent Data"], w321) -> (w316:string[])
          }
          event "Y.Scale.Auto": Value Change {
            n108 = event-data() -> ("NewVal"=w324:bool)  [unwired: 1 in]
            n109 = Bundle By Name(cluster=w326, "Persistent Data.Graph Props.Scale Properties.Y.Auto"=w324) -> (w325:T10)
            n110 = Build Array (concatenate)(string[] ["Set Autoscale Y", "Save Persistent Data"], w328) -> (w323:string[])
          }
          event "Legend": Value Change {
            # "Handle here since it is only set here"
            n111 = event-data() -> ("NewVal"=w336:bool)  [unwired: 1 in]
            n112 = Unbundle By Name(w331) -> ("References.Graph"=w330:refnum<vi>)
            n113 = Not(x=w336) -> (.not. x?=w329:bool)
            n114 = property on="Property Node" class="XYGraph (strict)"(reference=w330, error in=w333, "Legend Visible"=w329) -> (error out=w332:errorcluster)  [unwired: 1 out]
            n115 = Bundle By Name(cluster=w331, "Persistent Data.Graph Props.Legend:Visible"=w329) -> (w337:T10)
            n116 = Build Array (concatenate)("Save Persistent Data", w338) -> (w335:string[])
          }
          event "Y.Scale.Once": Value Change {
            # "Handle here since this can only be called by the button and it is not persistent"
            n117 = event-data() -> ()  [unwired: 1 in, 1 out]
            n118 = Unbundle By Name(w346) -> ("References.Graph"=w345:refnum<vi>)
            n119 = property on="Property Node" class="XYGraph (strict)"(reference=w345, error in=w348, "YScale.ScaleFit"=u8 1 ("X Scale.Scale Fit")) -> (error out=w347:errorcluster, "YScale.Maximum"=w340:dbl, "YScale.Minimum"=w339:dbl)  [unwired: 1 out]
            n120 = Build Array (concatenate)("Save Persistent Data", w349) -> (w343:string[])
            n121 = Bundle By Name(cluster=w346, "Persistent Data.Graph Props.Scale Properties.Y.Max"=w340, "Persistent Data.Graph Props.Scale Properties.Y.Min"=w339) -> (w341:T10)
          }
          event "X.Scale.Once": Value Change {
            # "Handle here since this can only be called by the button and it is not persistent"
            n122 = event-data() -> ()  [unwired: 1 in, 1 out]
            n123 = Unbundle By Name(w357) -> ("References.Graph"=w356:refnum<vi>)
            n124 = property on="Property Node" class="XYGraph (strict)"(reference=w356, error in=w359, "XScale.ScaleFit"=u8 1 ("X Scale.Scale Fit")) -> (error out=w358:errorcluster, "XScale.Maximum"=w351:dbl, "XScale.Minimum"=w350:dbl)  [unwired: 1 out]
            n125 = Build Array (concatenate)("Save Persistent Data", w360) -> (w354:string[])
            n126 = Bundle By Name(cluster=w357, "Persistent Data.Graph Props.Scale Properties.X.Max"=w351, "Persistent Data.Graph Props.Scale Properties.X.Min"=w350) -> (w352:T10)
          }
          event "Graph": Scale Range Change {
            # "User changed scale manually"
            n127 = event-data() -> ("Kind"=w361:enum16{"X-Scale", "Y-Scale", "Z-Scale"}, "NewRange.Minimum"=w364:dbl, "NewRange.Maximum"=w363:dbl)  [unwired: 1 in]
            n128 = case shown="\"Y-Scale\"" w361 {
              tunnel: w365 -> [w372 w377 w378]
              tunnel: w364 -> [w371 w376 _]
              tunnel: w363 -> [w370 w375 _]
              tunnel: [w369 w374 w378] -> w362
              frame "Y-Scale" {
                n129 = Bundle By Name(cluster=w372, "Persistent Data.Graph Props.Scale Properties.Y.Min"=w371, "Persistent Data.Graph Props.Scale Properties.Y.Max"=w370, "System.Save"=TRUE) -> (w369:T10)
              }
              frame "X-Scale" {
                n130 = Bundle By Name(cluster=w377, "Persistent Data.Graph Props.Scale Properties.X.Min"=w376, "Persistent Data.Graph Props.Scale Properties.X.Max"=w375, "System.Save"=TRUE) -> (w374:T10)
              }
              frame Default {
              }
            }
          }
          event "Graph": Shortcut Menu Selection? (App) {
            n131 = event-data() -> ("ItemTag"=w385:string)  [unwired: 1 in]
            n132 = case shown="\"APP_SC_IGNORE_TIME_STAMP\"" w385 {
              tunnel: [FALSE ("Discard?") TRUE ("Discard?") TRUE ("Discard?") TRUE ("Discard?")] -> w386
              tunnel: [w387 w399 w410 w420] -> w384
              tunnel: w383 -> [w387 w400 w411 w421]
              tunnel: w382 -> [w389 w401 w409 w419]
              tunnel: [w389 w397 w409 w419] -> w381
              tunnel: [w388 w392 w407 w417] -> w380
              tunnel: w379 -> [w388 w393 w407 w417]
              frame Default {
              }
              frame "APP_SC_IGNORE_TIME_STAMP" {
                n133 = Unbundle By Name(w401) -> ("References.Graph"=w398:refnum<vi>)
                n134 = property class="XYGraph (strict)"(reference=w398, error in=w400) -> (error out=w399:errorcluster, "IgnoreTimestamp"=w396:bool)  [unwired: 1 out]
                n135 = Not(x=w396) -> (.not. x?=w395:bool)
                n136 = Build Array (concatenate)(string[] ["Set X&Y Format & Precision", "Save Persistent Data"], w393) -> (w392:string[])
                n137 = Bundle By Name(cluster=w401, "Persistent Data.Graph Props.Scale Properties.X.IgnoreTS"=w395) -> (w397:T10)
              }
              frame "APP_SC_AUTOSCALE_Y" {
                # "reroute it like a button press"
                n138 = Unbundle By Name(w409) -> ("References.Y.Scale.Auto"=w406:refnum<vi>)
                n139 = property class="Bool (strict)"(reference=w406, error in=w411) -> (reference out=w404:refnum<vi>, error out=w405:errorcluster, "Value"=w403:bool)
                n140 = Not(x=w403) -> (.not. x?=w402:bool)
                n141 = property class="Bool (strict)"(reference=w404, error in=w405, "Val(Sgnl)"=w402) -> (error out=w410:errorcluster)  [unwired: 1 out]
              }
              frame "APP_SC_AUTOSCALE_X" {
                # "reroute it like a button press"
                n142 = Unbundle By Name(w419) -> ("References.X.Scale.Auto"=w416:refnum<vi>)
                n143 = property class="Bool (strict)"(reference=w416, error in=w421) -> (reference out=w414:refnum<vi>, error out=w415:errorcluster, "Value"=w413:bool)
                n144 = Not(x=w413) -> (.not. x?=w412:bool)
                n145 = property class="Bool (strict)"(reference=w414, error in=w415, "Val(Sgnl)"=w412) -> (error out=w420:errorcluster)  [unwired: 1 out]
              }
            }
            n146 = event-data("Discard?"=w386) -> ()  [unwired: 1 in, 1 out]
          }
        }
      }
      frame "Error" {
        n147 = Unbundle By Name(w426) -> ("System.ErrState"=w425:string)
        n148 = Unbundle By Name(w424) -> ("source"=w428:string)
        n149 = Concatenate Strings(w428, "<APPEND> State: " ("string"), w425) -> (w423:string)
        n150 = Bundle By Name(cluster=w424, "source"=w423) -> (w422:errorcluster)
        n151 = call "Simple Error Handler.vi"("error in (no error)"=w422) -> ()  [unwired: 4 in, 5 out]
      }
      frame "Save Persistent Data" {
        # "Instead of calling once at shut down, this is called often. Because by the time we are shutting down, it is too late to save data- The workspace isnt listening."
        n152 = Unbundle By Name(w433) -> ("Persistent Data"=w434:T13)
        n153 = call "XY Persistent Data to Variant.vi"("error in (no error)"=w436, "Persistent Data"=w434) -> ("error out"=w435:errorcluster, "Variant"=w431:variant)  [unwired: 8 in]
        n154 = Bundle By Name(cluster=w433, "Custom Data"=w431) -> (w432:T10)
        n155 = Unbundle By Name(w432) -> ("System.To Workspace"=w443:refnum<user-event>, "Custom Data"=w438:variant)
        n156 = Bundle By Name(cluster=T26 {"Operation"=enum."SetCustomData", "Data"=variant} ("event data"), "Operation"=enum16{"SetCustomData", "DeleteItem"}."SetCustomData", "Data"=w438) -> (w441:T26)
        n157 = Generate User Event(user event=w443, event data cluster=w441, error in=w435) -> (error out=w439:errorcluster)  [unwired: 1 in, 1 out]
      }
      frame "Check NonEvent Properties" {
        # "use this case to check any properties that don't have an event associated with them. for example, someone changing a legend text doesn't fire an event... but we still want to save that change"
        n158 = call "Check For XY Renamed Plots.vi"("error in (no error)"=w447, "Waveform Graph Data in"=w446) -> ("error out"=w444:errorcluster, "Waveform Graph Data out"=w445:T10)  [unwired: 8 in]
      }
      frame "LaunchConfigDialog" {
        n159 = call "Launch XY Config Dialog.vi"("error in (no error)"=w452, "Waveform Graph Data in"=w449) -> ("error out"=w451:errorcluster)  [unwired: 9 in]
      }
      frame "Validate Channels" {
        n160 = Unbundle By Name(w458) -> ("System.Root"=w456:refnum<k24>, "Persistent Data.UDP Data.Channel Paths"=w454:string[])
        n161 = call "Validate Channels.vi"("Channel Paths"=w454, "Root"=w456) -> ("Valid Channels?"=w455:bool)  [unwired: 9 in]
        n162 = Bundle By Name(cluster=w458, "System.Valid Channels?"=w455) -> (w457:T10)
      }
      frame "Delete" {
        n163 = Unbundle By Name(w467) -> ("System.To Workspace"=w465:refnum<user-event>)
        n164 = Bundle By Name(cluster=T26 {"Operation"=enum."DeleteItem", "Data"=variant} ("event data"), "Operation"=enum16{"SetCustomData", "DeleteItem"}."DeleteItem") -> (w462:T26)
        n165 = Generate User Event(user event=w465, event data cluster=w462, error in=w466) -> (error out=w464:errorcluster)  [unwired: 1 in, 1 out]
      }
      frame "<------------- UDP Streaming ------------->" {
      }
      frame "Change Update Rate" {
        n166 = Unbundle By Name(w481) -> ("System.Graph Update Queue"=w476:refnum<queue>, "Persistent Data.UDP Data.Update Rate"=w474:T20)
        n167 = Index Array(array=u32[] [67, 100, 200, 250, 333, 500, 1000, 2000], index=w474) -> (element=w471:u32)
        n168 = To Variant(anything=w471) -> (Variant=w478:variant)
        n169 = Bundle By Name(cluster=T8 {"Graph Update Action State"=enum."Active", "Data"=variant} ("notification"), "Graph Update Action State"=Graph_Update_Action_State."Change Rate", "Data"=w478) -> (w477:T8)
        n170 = Enqueue Element At Opposite End(queue=w476, element=w477, error in (no error)=w473) -> (error out=w472:errorcluster)  [unwired: 1 in, 2 out]
      }
      frame "<------------- Front Panel Updates------------->" {
      }
      frame "Set Label" {
        n171 = Unbundle By Name(w487) -> ("Persistent Data.Label"=→"Label":string)
      }
      frame "Set Autoscale X" {
        # "If autoscale was turned off, save the current range"
        # "Make sure the button value is consistent in case this was set at start up or by the dialog"
        n172 = Unbundle By Name(w499) -> ("References.X.Scale.Once"=w491:refnum<vi>, "References.X.Scale.Auto"=w501:refnum<vi>, "References.Graph"=w505:refnum<vi>, "Persistent Data.Graph Props.Scale Properties.X.Auto"=w493:bool)
        "X.Autoscale" <- w493
        n173 = Select(t=u8 2 ("X Scale.Scale Fit"), s=w493, f=u8 0 ("X Scale.Scale Fit")) -> (s? t:f=w502:u8)
        n174 = property on="Property Node" class="XYGraph (strict)"(reference=w505, error in=w506, "XScale.ScaleFit"=w502) -> (error out=w500:errorcluster, "XScale.Minimum"=w497:dbl, "XScale.Maximum"=w496:dbl)  [unwired: 1 out]
        n175 = Build Array(w491) -> (w490:refnum<vi>[])
        n176 = case shown="True" w493 {
          tunnel: w499 -> [w511 w512]
          tunnel: [w510 w512] -> w498
          tunnel: w497 -> [w509 _]
          tunnel: w496 -> [w508 _]
          frame False {
            n177 = Bundle By Name(cluster=w511, "Persistent Data.Graph Props.Scale Properties.X.Min"=w509, "Persistent Data.Graph Props.Scale Properties.X.Max"=w508) -> (w510:T10)
          }
          frame True {
          }
        }
        n178 = property on="Property Node" class="Bool (strict)"(reference=w501, error in=w500, "Value"=w493) -> (error out=w494:errorcluster)  [unwired: 1 out]
        n179 = Not(x=w493) -> (.not. x?=w492:bool)
        n180 = call "XY Set Control Enable State.vi"("error in (no error)"=w494, "Enabled?"=w492, "Controls"=w490) -> ("error out"=w495:errorcluster)  [unwired: 8 in]
      }
      frame "Set Autoscale Y" {
        # "If autoscale was turned off, save the current range"
        # "Make sure the button value is consistent in case this was set at start up or by the dialog"
        n181 = Unbundle By Name(w522) -> ("References.Y.Scale.Once"=w514:refnum<vi>, "References.Y.Scale.Auto"=w524:refnum<vi>, "References.Graph"=w528:refnum<vi>, "Persistent Data.Graph Props.Scale Properties.Y.Auto"=w515:bool)
        "Y.Autoscale" <- w515
        n182 = Select(t=u8 2 ("X Scale.Scale Fit"), s=w515, f=u8 0 ("X Scale.Scale Fit")) -> (s? t:f=w525:u8)
        n183 = property on="Property Node" class="XYGraph (strict)"(reference=w528, error in=w529, "YScale.ScaleFit"=w525) -> (error out=w523:errorcluster, "YScale.Minimum"=w520:dbl, "YScale.Maximum"=w519:dbl)  [unwired: 1 out]
        n184 = Build Array(w514) -> (w513:refnum<vi>[])
        n185 = case shown="True" w515 {
          tunnel: w522 -> [w534 w535]
          tunnel: [w533 w535] -> w521
          tunnel: w520 -> [w532 _]
          tunnel: w519 -> [w531 _]
          frame False {
            n186 = Bundle By Name(cluster=w534, "Persistent Data.Graph Props.Scale Properties.Y.Min"=w532, "Persistent Data.Graph Props.Scale Properties.Y.Max"=w531) -> (w533:T10)
          }
          frame True {
          }
        }
        n187 = property on="Property Node" class="Bool (strict)"(reference=w524, error in=w523, "Value"=w515) -> (error out=w518:errorcluster)  [unwired: 1 out]
        n188 = Not(x=w515) -> (.not. x?=w516:bool)
        n189 = call "XY Set Control Enable State.vi"("error in (no error)"=w518, "Enabled?"=w516, "Controls"=w513) -> ("error out"=w517:errorcluster)  [unwired: 8 in]
      }
      frame "Set BGColor" {
        n190 = Unbundle By Name(w539) -> ("References.Graph"=w538:refnum<vi>, "Persistent Data.Graph Props.BgColor"=w536:u32)
        n191 = property on="Property Node" class="XYGraph (strict)"(reference=w538, error in=w540, "BG Color"=w536) -> (error out=w537:errorcluster)  [unwired: 1 out]
      }
      frame "Set X&Y Format & Precision" {
        n192 = Unbundle By Name(w551) -> ("Persistent Data.Graph Props.Scale Properties.Y.Format"=w550:T18, "Persistent Data.Graph Props.Scale Properties.Y.Precision:"=w549:T17, "References.Graph"=w546:refnum<vi>, "Persistent Data.Graph Props.Scale Properties.X.Format"=w542:T18, "Persistent Data.Graph Props.Scale Properties.X.Precision"=w543:T17)
        n193 = case shown="Default" w542 {
          selector: w542 -> [w555 _]
          tunnel: w547 -> [w558 w562]
          tunnel: w546 -> [w557 w561]
          tunnel: [w556 w563] -> w544
          tunnel: w543 -> [w554 _]
          tunnel: [w553 w559] -> w545
          frame Default {
            n194 = property on="Property Node" class="XYGraph (strict)"(reference=w557, error in=w558, "XScale.Format"=w555, "XScale.Precision"=w554) -> (reference out=w553:refnum<vi>, error out=w556:errorcluster)
          }
          frame 9 {
            # "9: Auto format is not writable. Rather it means a format string is applied"
            n195 = property on="Property Node" class="XYGraph (strict)"(reference=w561, error in=w562, "XScale.FormatString"="%#_g" ("X Scale.Format String")) -> (reference out=w559:refnum<vi>, error out=w563:errorcluster)
          }
        }
        n196 = case shown="Default" w550 {
          selector: w550 -> [w565 _]
          tunnel: w544 -> [w568 w571]
          tunnel: w545 -> [w567 w570]
          tunnel: [w566 w572] -> w548
          tunnel: w549 -> [w564 _]
          frame Default {
            n197 = property on="Property Node" class="XYGraph (strict)"(reference=w567, error in=w568, "YScale.Format"=w565, "YScale.Precision"=w564) -> (error out=w566:errorcluster)  [unwired: 1 out]
          }
          frame 9 {
            # "9: Auto format is not writable. Rather it means a format string is applied"
            n198 = property on="Property Node" class="XYGraph (strict)"(reference=w570, error in=w571, "YScale.FormatString"="%#_g" ("X Scale.Format String")) -> (error out=w572:errorcluster)  [unwired: 1 out]
          }
        }
      }
      frame "Set X&Y Max & Min" {
        # "Dont set range if auto scale is on."
        n199 = Unbundle By Name(w583) -> ("References.Graph"=w582:refnum<vi>, "Persistent Data.Graph Props.Scale Properties.X.Auto"=w577:bool, "Persistent Data.Graph Props.Scale Properties.X.Max"=w581:dbl, "Persistent Data.Graph Props.Scale Properties.X.Min"=w580:dbl, "Persistent Data.Graph Props.Scale Properties.Y.Auto"=w575:bool, "Persistent Data.Graph Props.Scale Properties.Y.Max"=w574:dbl, "Persistent Data.Graph Props.Scale Properties.Y.Min"=w573:dbl)
        n200 = case shown="False" w577 {
          tunnel: w584 -> [w597 w598]
          tunnel: w582 -> [w596 w599]
          tunnel: w581 -> [w595 _]
          tunnel: w580 -> [w594 _]
          tunnel: [w593 w598] -> w579
          tunnel: [w592 w599] -> w578
          frame False {
            n201 = property on="Property Node" class="XYGraph (strict)"(reference=w596, error in=w597, "XScale.Maximum"=w595, "XScale.Minimum"=w594) -> (reference out=w592:refnum<vi>, error out=w593:errorcluster)
          }
          frame True {
          }
        }
        n202 = case shown="False" w575 {
          tunnel: w579 -> [w590 w591]
          tunnel: w578 -> [w589 _]
          tunnel: [w588 w591] -> w576
          tunnel: w574 -> [w587 _]
          tunnel: w573 -> [w586 _]
          frame False {
            n203 = property on="Property Node" class="XYGraph (strict)"(reference=w589, error in=w590, "YScale.Maximum"=w587, "YScale.Minimum"=w586) -> (error out=w588:errorcluster)  [unwired: 1 out]
          }
          frame True {
          }
        }
      }
      frame "Set Axis Labels" {
        n204 = Unbundle By Name(w617) -> ("System.Root"=w600:refnum<k24>, "Persistent Data.UDP Data.Channel Paths"=w605:string[], "Persistent Data.UDP Data.Channel Names"=w602:string[], "References.Graph"=w616:refnum<vi>, "Persistent Data.Graph Props.Scale Properties.X.DefLabel"=w612:bool, "Persistent Data.Graph Props.Scale Properties.X.Label:"=w611:string, "Persistent Data.Graph Props.Scale Properties.X.LabelVis"=w613:bool, "Persistent Data.Graph Props.Scale Properties.Y.DefLabel"=w608:bool, "Persistent Data.Graph Props.Scale Properties.Y.Label:"=w607:string, "Persistent Data.Graph Props.Scale Properties.Y.LabelVis"=w610:bool)
        n205 = Index Array(array=w605) -> (element=w603:string)  [unwired: 1 in]
        n206 = Index Array(array=w602) -> (element=w601:string)  [unwired: 1 in]
        n207 = Select(t="Amplitude", s=w608, f=w607) -> (s? t:f=w606:string)
        n208 = call "Get Channel Name.vi"("Channel Name"=w601, "Channel Path"=w603, "Root"=w600) -> ("Name"=w604:string)  [unwired: 8 in]
        n209 = Select(t=w604, s=w612, f=w611) -> (s? t:f=w614:string)
        n210 = property on="Property Node" class="XYGraph (strict)"(reference=w616, error in=w618, "XScale.NameLbl.Text"=w614, "XScale.NameLbl.Visible"=w613, "YScale.NameLbl.Text"=w606, "YScale.NameLbl.Visible"=w610) -> (error out=w615:errorcluster)  [unwired: 1 out]
      }
      frame "Set Legend" {
        n211 = Unbundle By Name(w634) -> ("System.Root"=w620:refnum<k24>, "Persistent Data.UDP Data.Channel Paths"=w626:string[], "Persistent Data.UDP Data.Channel Names"=w622:string[], "References.Graph"=w628:refnum<vi>, "Persistent Data.Graph Props.Legend:Visible"=w627:bool)
        n212 = Array Subset(array=w626, index=1) -> (w625:string[])  [unwired: 1 in]
        n213 = Array Subset(array=w622, index=1) -> (w621:string[])  [unwired: 1 in]
        n214 = Array Size(array=w625) -> (size(s)=w630:i32)
        n215 = property class="XYGraph (strict)"(reference=w628, error in=w632, "LegNumRows"=w630, "Legend Visible"=w627) -> (reference out=w629:refnum<vi>, error out=w631:errorcluster)
        n216 = case shown="Default" w630 {
          tunnel: [w641 w655] -> w633
          tunnel: w631 -> [w640 w651]
          tunnel: w625 -> [w639 _]
          tunnel: w629 -> [w638 w652]
          tunnel: w621 -> [w637 _]
          tunnel: w620 -> [w636 _]
          frame Default {
            n217 = for {
              shift-right: [w648] -> w641
              shift-left: w640 -> [w649]
              tunnel: w639 -> [w645] mode=indexing
              tunnel: w638 -> [w646]
              tunnel: w637 -> [w643] mode=indexing
              tunnel: w636 -> [w642]
              i -> [w647]
              n218 = call "Get Channel Name.vi"("Channel Name"=w643, "Channel Path"=w645, "Root"=w642) -> ("Name"=w644:string)  [unwired: 8 in]
              n219 = property class="XYGraph (strict)"(reference=w646, error in=w649, "Active Plot"=w647, "Plot.Plot Name"=w644) -> (error out=w648:errorcluster)  [unwired: 1 out]
            }
          }
          frame 0 {
            # "If there are no streams this is a good opportunity to clear the graph"
            n220 = property class="XYGraph (strict)"(reference=w652, error in=w651, "Active Plot"=u32 0, "Plot.Plot Name"="Plot 0", "Value"=cluster{"X":dbl[], "Y":dbl[]}[] []) -> (error out=w655:errorcluster)  [unwired: 1 out]
          }
        }
      }
      frame "<------------------ Shut Down ------------------>" {
      }
      frame "Delete Events" {
        # "These nodes run even if error occures"
        n221 = Unbundle By Name(w684) -> ("System.ToDialog"=w668:refnum<user-event>, "System.DialogEventReg"=w670:refnum<event-registration>, "System.Update Graph"=w661:refnum<user-event>, "System.Periodic"=w671:refnum<user-event>, "System.FromDialog"=w675:refnum<user-event>, "System.To Workspace"=w682:refnum<user-event>, "System.From Workspace"=w683:refnum<user-event>, "EventRegs.Graph"=w680:refnum<event-registration>, "System.SystemStateRefs"=w677:T22, "System.Graph Update Queue"=w664:refnum<queue>, "System.UDP Queue"=w663:refnum<queue>)
        n222 = call "NI VeriStand - Close Engine State Change Notification.vi"("SystemStateRefs"=w677) -> ("error out"=w673:errorcluster)  [unwired: 10 in]
        n223 = Release Queue(queue=w664) -> (error out=w665:errorcluster)  [unwired: 2 in, 2 out]
        n224 = Release Queue(queue=w663) -> (error out=w662:errorcluster)  [unwired: 2 in, 2 out]
        n225 = Unregister For Events(event registration refnum=w680) -> (error out=w679:errorcluster)  [unwired: 1 in]
        n226 = Destroy User Event(user event=w683, error in=w679) -> (error out=w678:errorcluster)
        n227 = Destroy User Event(user event=w682, error in=w678) -> (error out=w676:errorcluster)
        n228 = Destroy User Event(user event=w675, error in=w676) -> (error out=w672:errorcluster)
        n229 = Destroy User Event(user event=w671, error in=w672) -> (error out=w659:errorcluster)
        n230 = Destroy User Event(user event=w661, error in=w659) -> (error out=w660:errorcluster)
        n231 = Unregister For Events(event registration refnum=w670) -> (error out=w669:errorcluster)  [unwired: 1 in]
        n232 = Destroy User Event(user event=w668, error in=w669) -> (error out=w666:errorcluster)
        n233 = Merge Errors(w667, w666, w660, w673, w665, w662) -> (w674:errorcluster)
      }
      frame "Close Managers" {
        # "These nodes run even if error occures"
        n234 = Unbundle By Name(w687) -> ("System.Workspace"=w686:T21)
        n235 = call "NI VeriStand - Close Workspace Manager Reference.vi"("error in (no error)"=w688, "WorkspaceManager"=w686) -> ("error out"=w685:errorcluster)  [unwired: 9 in]
      }
      frame "Wait for NIVS Helper" {
        # "This node runs even if error occures"
        # "Wait for the NIVS helper VI to finish"
        n236 = Unbundle By Name(w698) -> ("System.NIVS helper"=w697:refnum<vi>)
        n237 = call-by-ref "Wait On Asynchronous Call"(reference=w697) -> (reference out=w693:refnum<vi>, error out=w696:errorcluster, 19:"error out"=w695:errorcluster)  [unwired: 20 in]
        n238 = Merge Errors(w696, w695) -> (w694:errorcluster)
        n239 = Close Reference(reference=w693, error in (no error)=w694) -> (error out=w690:errorcluster)
        n240 = Merge Errors(w692, w690) -> (w691:errorcluster)
      }
      frame "Exit" {
      }
      frame "<------------------ Macros ------------------>" {
      }
      frame "MACRO - Initialize" {
        # "Save persistent data at the end so we can detect if this control is new or not after next load"
        n241 = Build Array (concatenate)(string[] ["Open Managers", "Create Events", "Get Control References", "Get Persistent Data", "Validate Channels", "Check Connection", "Initialize Plots & Legend", "MACRO - Refresh Graph", "Launch NIVS Helper", "Save Persistent Data"], w708) -> (w707:string[])
      }
      frame "MACRO - Shut Down" {
        n242 = Build Array (concatenate)(string[] ["Delete Events", "Close Managers", "Wait for NIVS Helper", "Exit"], w715) -> (w714:string[])
      }
      frame "MACRO - Refresh Graph" {
        n243 = Build Array (concatenate)(string[] ["Change Update Rate", "Set Label", "Set X&Y Max & Min", "Set Autoscale X", "Set Autoscale Y", "Set BGColor", "Set X&Y Format & Precision", "Set Axis Labels", "Set Legend"], w721) -> (w718:string[])
      }
      frame "MACRO - Disconnect" {
        n244 = Build Array (concatenate)(string[] ["Close UDP Streaming"], w724) -> (w723:string[])
      }
      frame "MACRO - System Disconnect" {
        n245 = Build Array (concatenate)(string[] ["System Close UDP Streaming"], w729) -> (w728:string[])
      }
      frame "MACRO - Connect" {
        n246 = Build Array (concatenate)(string[] ["Save Persistent Data", "Change Update Rate", "Open UDP Streaming"], w736) -> (w733:string[])
      }
      frame "<----------------- Disconnect ------------------->" {
      }
      frame "Close UDP Streaming" {
        n247 = Unbundle By Name(w751) -> ("System.UDPChannelStreamSession"=w745:T23, "System.Graph Update Queue"=w753:refnum<queue>, "System.UDP Queue"=w754:refnum<queue>)
        n248 = Enqueue Element(queue=w754, element=T9 {"UDP Action State"=enum."Close", "Data"=variant} ("notification"), error in (no error)=w752) -> (error out=w744:errorcluster)  [unwired: 1 in, 2 out]
        n249 = Enqueue Element(queue=w753, element=T8 {"Graph Update Action State"=enum."Inactive", "Data"=variant} ("notification"), error in (no error)=w744) -> (error out=w743:errorcluster)  [unwired: 1 in, 2 out]
        n250 = call "NI VeriStand - Undeploy UDP Channel Streaming Session.vi"("error in (no error)"=w743, "UDPChannelStreamSession in"=w745) -> ("error out"=w742:errorcluster, "UDPChannelStreamSession out"=w740:T23)  [unwired: 8 in]
        n251 = Bundle By Name(cluster=w751, "UDP Stream Active?"=FALSE, "System.UDPChannelStreamSession"=T23 refnum) -> (w750:T10)
        n252 = call "NI VeriStand - Close UDP Channel Streaming Session.vi"("error in (no error)"=w742, "UDPChannelStreamSession in"=w740) -> ("error out"=w741:errorcluster)  [unwired: 9 in]
      }
      frame "System Close UDP Streaming" {
        n253 = Unbundle By Name(w765) -> ("System.UDPChannelStreamSession"=w757:T23, "System.Graph Update Queue"=w767:refnum<queue>, "System.UDP Queue"=w768:refnum<queue>)
        n254 = Enqueue Element(queue=w768, element=T9 {"UDP Action State"=enum."Close", "Data"=variant} ("notification"), error in (no error)=w766) -> (error out=w759:errorcluster)  [unwired: 1 in, 2 out]
        n255 = Enqueue Element(queue=w767, element=T8 {"Graph Update Action State"=enum."Inactive", "Data"=variant} ("notification"), error in (no error)=w759) -> (error out=w756:errorcluster)  [unwired: 1 in, 2 out]
        n256 = Bundle By Name(cluster=w765, "UDP Stream Active?"=FALSE, "System.UDPChannelStreamSession"=T23 refnum) -> (w764:T10)
        n257 = call "NI VeriStand - Close UDP Channel Streaming Session.vi"("error in (no error)"=w756, "UDPChannelStreamSession in"=w757) -> ("error out"=w758:errorcluster)  [unwired: 9 in]
      }
      frame "<----------------- Connect ------------------->" {
      }
      frame "Open UDP Streaming" {
        n258 = Unbundle By Name(w791) -> ("System.Workspace"=w795:T21, "System.Graph Update Queue"=w786:refnum<queue>, "System.UDP Queue"=w789:refnum<queue>, "Persistent Data.UDP Data"=w774:T19, "System.Root"=w788:refnum<k24>, "Persistent Data.UDP Data.History Length"=w785:dbl, "Persistent Data.UDP Data.Decimation"=w783:i32)
        n259 = call "Get UDP Buffer Size.vi"("Decimation"=w783, "History Length"=w785, "Root"=w788) -> ("Buffer Size"=w782:i32)  [unwired: 8 in]
        n260 = call "Init UDP Config.vi"("error in (no error)"=w794, "Graph Buffer Size"=w782, "UDP Data"=w774, "Workspace anager in"=w795) -> ("error out"=w779:errorcluster, "UDP Stream Configuration"=w776:T5, "UDPChannelStreamSession out"=w792:T23, "WorkspaceManager out"=w793:T21)  [unwired: 4 in]
        n261 = To Variant(anything=w776) -> (Variant=w775:variant)
        n262 = Bundle By Name(cluster=T9 {"UDP Action State"=enum."Idle", "Data"=variant} ("notification"), "UDP Action State"=UDP_Action_State."Open", "Data"=w775) -> (w777:T9)
        n263 = Enqueue Element(queue=w789, element=w777, error in (no error)=w779) -> (error out=w784:errorcluster)  [unwired: 1 in, 2 out]
        n264 = Bundle By Name(cluster=w791, "System.Workspace"=w793, "System.UDPChannelStreamSession"=w792, "UDP Stream Active?"=TRUE) -> (w790:T10)
        n265 = Enqueue Element(queue=w786, element=T8 {"Graph Update Action State"=enum."Active", "Data"=variant} ("notification"), error in (no error)=w784) -> (error out=w787:errorcluster)  [unwired: 1 in, 2 out]
      }
      frame "<------------------ Initialization ------------------>" {
      }
      frame "Open Managers" {
        n266 = Unbundle By Name(w802) -> ("System.Gtwy"=w801:string)
        n267 = call "NI VeriStand - Open Workspace Manager Reference.vi"("error in (no error)"=w805, "Gateway IP Address (\"\": localhost)"=w801) -> ("error out"=w800:errorcluster, "WorkspaceManager"=w803:T21)  [unwired: 8 in]
        n268 = Bundle By Name(cluster=w802, "System.Workspace"=w803) -> (w804:T10)
      }
      frame "Create Events" {
        n269 = call "Create XY Events.vi"("error in (no error)"=w808, "Waveform Graph Data in"=w807) -> ("error out"=w810:errorcluster, "Waveform Graph Data out"=w811:T10)  [unwired: 8 in]
      }
      frame "Get Control References" {
        n270 = control-ref of="Graph"() -> (w812:refnum<vi>)
        n271 = control-ref of="X.Scale.Auto"() -> (w816:refnum<vi>)
        n272 = control-ref of="Y.Scale.Auto"() -> (w817:refnum<vi>)
        n273 = control-ref of="X.Scale.Once"() -> (w815:refnum<vi>)
        n274 = control-ref of="Y.Scale.Once"() -> (w814:refnum<vi>)
        n275 = control-ref of="Legend"() -> (w813:refnum<vi>)
        n276 = Bundle By Name(cluster=w820, "References.Graph"=w812, "References.X.Scale.Auto"=w816, "References.Y.Scale.Auto"=w817, "References.X.Scale.Once"=w815, "References.Y.Scale.Once"=w814, "References.LegendVis"=w813) -> (w819:T10)
      }
      frame "Get Persistent Data" {
        # "True if this is a brand new control. Used by the from workspace event"
        n277 = Unbundle By Name(w829) -> ("Custom Data"=w830:variant)
        n278 = call "XY Variant to Persistent Data.vi"("error in (no error)"=w832, "Variant"=w830) -> ("error out"=w831:errorcluster, "Persistent Data"=w822:T13, "New"=w826:bool)  [unwired: 7 in]
        n279 = Build Array (concatenate)("Initialize Dialog", w827) -> (w824:string[])
        n280 = Select(t=w824, s=w826, f=w827) -> (s? t:f=w823:string[])
        n281 = Bundle By Name(cluster=w829, "System.New"=w826, "Persistent Data"=w822) -> (w828:T10)
      }
      frame "Initialize Dialog" {
        n282 = Bundle By Name(cluster=w836, "Persistent Data.UDP Data"=T19 {"Decimation"=1, "UDP Buffer Size"=8192, "History Length"=10.0, "Update Rate"=enum."5 Hz", "Channel Paths"=[], "Channel Names"=[]}, "System.Valid Channels?"=FALSE) -> (w835:T10)
      }
      frame "Check Connection" {
        w848 = T30 1 items=["Idle", "Active"] ("x")
        # "This only needs to be done at start up because while running we will get the system state change event"
        n283 = Unbundle By Name(w842) -> ("System.Valid Channels?"=w839:bool, "System.Workspace"=w850:T21)
        n284 = call "NI VeriStand - Get System State.vi"("error in (no error)"=w852, "WorkspaceManager in"=w850) -> ("error out"=w851:errorcluster, "System State"=w849:T30)  [unwired: 5 in, 3 out]
        n285 = Equal?(x=w848, y=w849) -> (x = y?=w840:bool)
        n286 = Bundle By Name(cluster=w842, "System.Connected?"=w840) -> (w843:T10)
        n287 = And(x=w839, y=w840) -> (x .and. y?=w841:bool)
        n288 = case shown="True" w841 {
          tunnel: [w854 w860] -> w847
          tunnel: w846 -> [w854 w859]
          tunnel: "MACRO - Connect" -> [_ w858]
          tunnel: [w853 w855] -> w844
          tunnel: w843 -> [w853 w857]
          frame False {
          }
          frame True {
            # "If we are connecting at start up... use the plot width that we last saved. This prevents weird behavior because NIVS might be resizing our widget  during workspace initialization."
            n289 = Bundle By Name(cluster=w857, "System.UseSavedWidth"=TRUE) -> (w855:T10)
            n290 = Build Array (concatenate)(w858, w859) -> (w860:string[])
          }
        }
      }
      frame "Initialize Plots & Legend" {
        n291 = Unbundle By Name(w870) -> ("References.LegendVis"=w864:refnum<vi>, "Persistent Data.Graph Props.Legend:Visible"=w863:bool, "References.Graph"=w861:refnum<vi>, "Persistent Data.Graph Props.Plots"=w868:T15[], "Persistent Data.Graph Props.Legend:Number of Rows"=w867:u32)
        n292 = call "Update XY Plots.vi"("error in (no error)"=w869, "Persistent Data.Graph Props.Legend:Number of Rows"=w867, "Plots"=w868, "Graph"=w861) -> ("error out"=w866:errorcluster)  [unwired: 7 in]
        n293 = Not(x=w863) -> (.not. x?=w862:bool)
        n294 = property class="Bool (strict)"(reference=w864, error in=w866, "Value"=w862) -> (error out=w865:errorcluster)  [unwired: 1 out]
      }
      frame "Launch NIVS Helper" {
        # "This VI is required to be run to connect this workspace object to the workspace. This VI will continue to run until this control is deleted or the workspace is closed. Therefore, launch it asynchronously so there is no need for a separate loop."
        n295 = Unbundle By Name(w879) -> ("System.From Workspace"=w877:refnum<user-event>, "System.To Workspace"=w876:refnum<user-event>)
        n296 = vi-ref "sub_Display Template Handler Custom.vi"() -> (w884:refnum<vi>)
        n297 = property class="VI"(reference=w884, error in=w885) -> (error out=w883:errorcluster, "Name"=w882:string)  [unwired: 1 out]
        n298 = Current VI's Path() -> (path=w878:path)
        n299 = Open VI Reference(type specifier VI Refnum (for type only)=refnum<vi> refnum, vi path=w882, options=256, error in (no error)=w883) -> (vi reference=w880:refnum<vi>, error out=w887:errorcluster)  [unwired: 2 in]
        n300 = call-by-ref "Start Asynchronous Call"(reference=w880, error in=w887, "Parent.Path"=w878, "ToWidgetEvent"=w877, "ToWorkspace"=w876, "Item.Data"=w875, "Resizable"=TRUE) -> (reference out=w872:refnum<vi>, error out=w886:errorcluster)  [unwired: 14 in, 1 out]
        n301 = Bundle By Name(cluster=w879, "System.NIVS helper"=w872) -> (w873:T10)
      }
    }
    n302 = Unbundle By Name(w122) -> ("System.ErrFlag"=w121:bool)
    n303 = Compound Arithmetic op=AND(invert w121, w119) -> (w120:bool)
    n304 = case shown="True" w120 {
      selector: w120 -> [_ w136]
      tunnel: w129 -> [w134 w139]
      tunnel: [w134 w140] -> w126
      tunnel: [w133 w137] -> w123
      tunnel: w122 -> [w133 w138]
      tunnel: w118 -> [_ w135]
      frame False {
      }
      frame True {
        n305 = Bundle By Name(cluster=w138, "System.ErrState"=w135, "System.ErrFlag"=w136) -> (w137:T10)
        n306 = Build Array (concatenate)("Error", w139) -> (w140:string[])
      }
    }
  }
